vi "sendValue.vi"(8 "error in (no error)":errorcluster, 10 "data":variant, 11 "startScanDt in":refnum<class "startScanDt.lvclass">) -> (0 "error out":errorcluster, 2 "function return":i32, 3 "startScanDt out":refnum<class "startScanDt.lvclass">)   [LabVIEW 2016, in "SALLV_MtAtElectrometer_Messaging.lvlib" / "startScanDt.lvclass"]
uses:
  startScanDt.lvclass
  ts_sallv_MtAtElectrometer/DataTypes/command_startScanDt.ctl
  ts_sallv_MtAtElectrometer/SALLV_MtAtElectrometer.lvlib
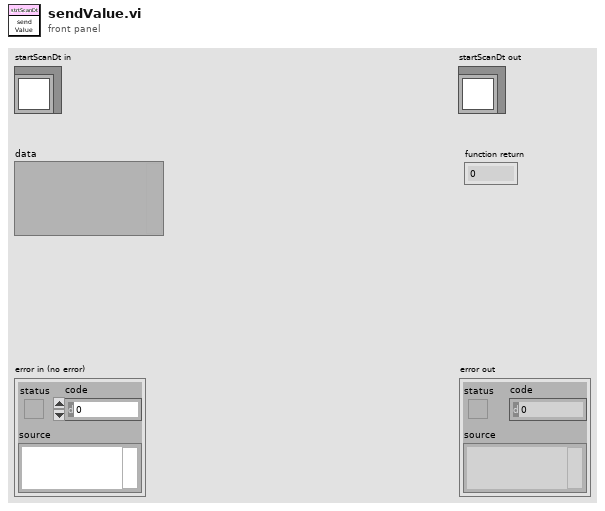
[diagram p1: front panel]
types:
  T1 = typedef "SALLV_MtAtElectrometer.lvlib/command_startScanDt.ctl" = cluster{"scanDuration":sgl}
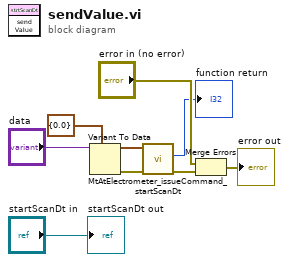
[diagram p0: block diagram]
diagram:
  n1 = Variant To Data(type=T1 {"scanDuration"=0.0} ("command_startScanDt_Ctl"), Variant="data") -> (data=w2:T1, error out=w5:errorcluster)  [unwired: 1 in]
  n2 = call "MtAtElectrometer_issueCommand_startScanDt.vi"("error in (no error)"=w5, "command_startScanDt_Ctl"=w2) -> ("error out"=w4:errorcluster, "function return"=→"function return":i32)  [unwired: 7 in, 1 out]
  n3 = Merge Errors("error in (no error)", w4) -> (→"error out":errorcluster)
  "startScanDt out" <- "startScanDt in"
